vi "Reference Position.vi"(6 "Size":refnum<class "Size.lvclass"> caption="Size (Unchanged)", 8 "error in (no error)":errorcluster, 9 "Offset":refnum<class "Offset.lvclass"> caption="Offset (None)", 10 "Alignment":T1={"Horizontal"=enum."Center", "Vertical"=enum."Center"} caption="Alignment (Center, Center)", 11 "Reference Position in":refnum<class "Reference Position.lvclass">) -> (0 "error out":errorcluster, 3 "Reference Position out":refnum<class "Reference Position.lvclass">)   [LabVIEW 2023, in "Panel Actor.lvlib" / "Panel.lvlib" / "Reference Position.lvclass"]
doc: "Constructs the Reference Position object.\n\n----\nPlease see the following web address for additional documentation and tutorial information:\nhttp://www.mooregoodideas.com/mgi-panel-manager/\n\nAuthor: Derek Trepanier\n\nCopyright (c) 2018, Moore Good Ideas, Inc.\n\nAll rights reserved.\n\nRedistribution and use in source and binary forms, with or without modification, are permitted provided that the following conditions are met:\n\n * Redistributions of source code must retain the above copyright notice, this list of conditions and the following disclaimer.\n * Redistributions in binary form must reproduce the above copyright notice, this list of conditions and the following disclaimer in the documentation and/or other materials provided with the distribution.\n * Neither the name of Moore Good Ideas, Inc. nor the names of its contributors may be used to endorse or promote products derived from this software without specific prior written permission.\n\nTHIS SOFTWARE IS PROVIDED BY THE COPYRIGHT HOLDERS AND CONTRIBUTORS \"AS IS\" AND ANY EXPRESS OR IMPLIED WARRANTIES, INCLUDING, BUT NOT LIMITED TO, THE IMPLIED WARRANTIES OF MERCHANTABILITY AND FITNESS FOR A PARTICULAR PURPOSE ARE DISCLAIMED. IN NO EVENT SHALL THE COPYRIGHT OWNER OR CONTRIBUTORS BE LIABLE FOR ANY DIRECT, INDIRECT, INCIDENTAL, SPECIAL, EXEMPLARY, OR CONSEQUENTIAL DAMAGES (INCLUDING, BUT NOT LIMITED TO, PROCUREMENT OF SUBSTITUTE GOODS OR SERVICES; LOSS OF USE, DATA, OR PROFITS; OR BUSINESS INTERRUPTION) HOWEVER CAUSED AND ON ANY THEORY OF LIABILITY, WHETHER IN CONTRACT, STRICT LIABILITY, OR TORT (INCLUDING NEGLIGENCE OR OTHERWISE) ARISING IN ANY WAY OUT OF THE USE OF THIS SOFTWARE, EVEN IF ADVISED OF THE POSSIBILITY OF SUCH DAMAGE."
uses:
  Reference Position.lvclass
  Alignment.ctl
  Horizontal Alignment.ctl
  Vertical Alignment.ctl
  Offset/Offset.lvclass
  Size/Size.lvclass
  Reference Position.lvclass/Reference Position.ctl
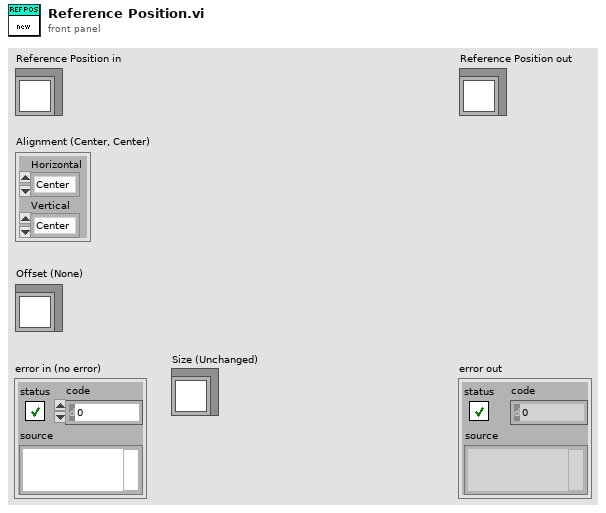
[diagram p1: front panel]
types:
  T1 = typedef "Panel Actor.lvlib/Panel.lvlib/Reference Position.lvclass/Alignment.ctl" = cluster{"Horizontal":T2, "Vertical":T3}
  T2 = typedef "Panel Actor.lvlib/Panel.lvlib/Reference Position.lvclass/Horizontal Alignment.ctl" = enum16{"Left", "Center", "Right"}
  T3 = typedef "Panel Actor.lvlib/Panel.lvlib/Reference Position.lvclass/Vertical Alignment.ctl" = enum16{"Top", "Center", "Bottom"}
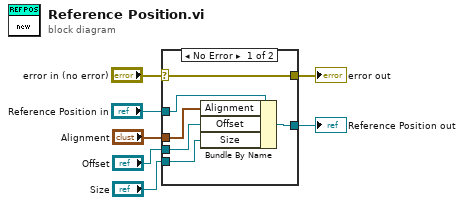
[diagram p0: block diagram]
diagram:
  n1 = case shown="No Error" "error in (no error)" {
    selector: "error in (no error)" -> [w12 w15]
    tunnel: [w12 w15] -> w6
    tunnel: [w11 w14] -> w4
    tunnel: "Reference Position in" -> [w13 w14]
    tunnel: "Alignment" -> [w10 _]
    tunnel: "Offset" -> [w9 _]
    tunnel: "Size" -> [w8 _]
    frame No Error {
      n2 = Bundle By Name(cluster=w13, "Alignment"=w10, "Offset"=w9, "Size"=w8) -> (w11:refnum<class "Reference Position.lvclass">)
    }
    frame Error {
    }
  }
  "error out" <- w6
  "Reference Position out" <- w4
